vi "update.vi"(8 "error in (no error)":errorcluster, 10 "model":refnum<class "Model.lvclass">, 11 "EnabledState in":refnum<class "EnabledState.lvclass">) -> (0 "error out":errorcluster, 2 "model 2":refnum<class "Model.lvclass">, 3 "EnabledState out":refnum<class "EnabledState.lvclass">)   [LabVIEW 2013, in "EnabledState.lvclass"]
uses:
  EnabledState.lvclass
  Model/Model/Model.lvclass
  Typedefs/StateSelector.ctl
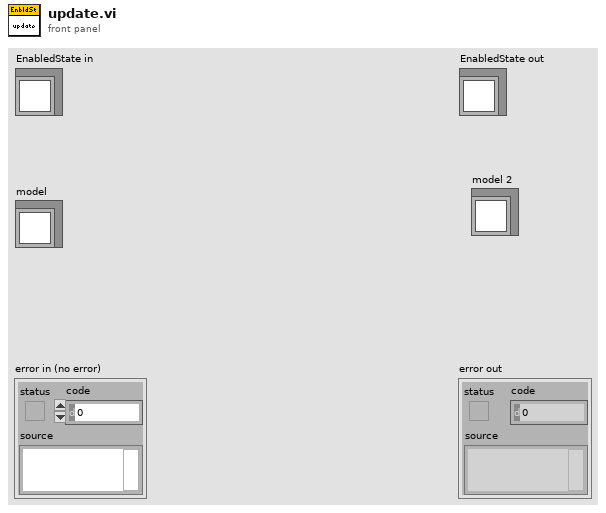
[diagram p1: front panel]
types:
  T1 = typedef "StateSelector.ctl" = enum16{"EndingCycleState", "FaultState", "InteractiveMotionState", "MovingToNewForceState", "OffState", "PausingState", "StandbyState", "StoppedState"}
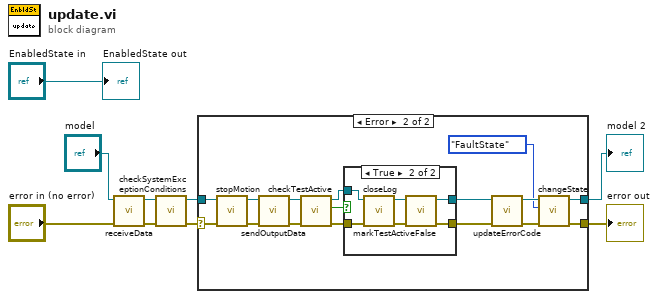
[diagram p0: block diagram]
diagram:
  n1 = call "receiveData.vi"("error in (no error)"="error in (no error)", "Model in"="model") -> ("error out"=w1:errorcluster, "Model out"=w3:refnum<class "Model.lvclass">)  [unwired: 8 in]
  n2 = call "checkSystemExceptionConditions.vi"("error in (no error)"=w1, "Model in"=w3) -> ("error out"=w6:errorcluster, "Model out"=w5:refnum<class "Model.lvclass">)  [unwired: 8 in]
  n3 = case shown="Error" w6 {
    selector: w6 -> [w11 w21]
    tunnel: [w11 w25] -> w9
    tunnel: w5 -> [w10 w22]
    tunnel: [w10 w24] -> w7
    frame No Error {
    }
    frame Error {
      n4 = call "stopMotion.vi"("error in (no error)"=w21, "Model in"=w22) -> ("error out"=w13:errorcluster, "Model out"=w15:refnum<class "Model.lvclass">)  [unwired: 8 in]
      n5 = call "sendOutputData.vi"("error in (no error)"=w13, "Model in"=w15) -> ("error out"=w12:errorcluster, "Model out"=w14:refnum<class "Model.lvclass">)  [unwired: 8 in]
      n6 = call "checkTestActive.vi"("error in (no error)"=w12, "Model in"=w14) -> ("error out"=w18:errorcluster, "testActiveIsTrue"=w20:bool, "Model out"=w19:refnum<class "Model.lvclass">)  [unwired: 7 in]
      n7 = case shown="True" w20 {
        tunnel: [w29 w32] -> w16
        tunnel: [w28 w30] -> w17
        tunnel: w19 -> [w29 w35]
        tunnel: w18 -> [w28 w34]
        frame False {
        }
        frame True {
          n8 = call "closeLog.vi"("error in (no error)"=w34, "Model in"=w35) -> ("error out"=w31:errorcluster, "Model out"=w33:refnum<class "Model.lvclass">)  [unwired: 8 in]
          n9 = call "markTestActiveFalse.vi"("error in (no error)"=w31, "Model in"=w33) -> ("error out"=w30:errorcluster, "Model out"=w32:refnum<class "Model.lvclass">)  [unwired: 8 in]
        }
      }
      n10 = call "updateErrorCode.vi"("error in (no error)"=w17, "Model in"=w16) -> ("error out"=w26:errorcluster, "Model out"=w27:refnum<class "Model.lvclass">)  [unwired: 8 in]
      n11 = call "changeState.vi"("error in (no error)"=w26, "State:"=StateSelector."FaultState", "Model in"=w27) -> ("error out"=w25:errorcluster, "Model out"=w24:refnum<class "Model.lvclass">)  [unwired: 7 in]
    }
  }
  "error out" <- w9
  "model 2" <- w7
  "EnabledState out" <- "EnabledState in"
